vi "User Event Handle.vi"(8 "error in":errorcluster, 10 "Array 2":bool[](array[boolean])) -> (0 "error out":errorcluster)   [LabVIEW 2016]
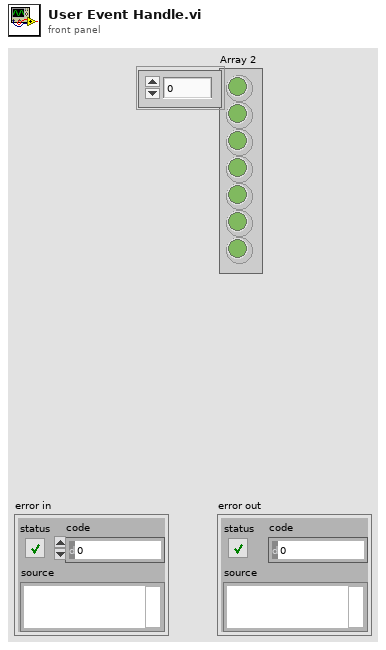
[diagram p1: front panel]
types:
  T1 = enum16{"Open", "Enqueue", "InsertQueue", "Release Queue", "Close"}
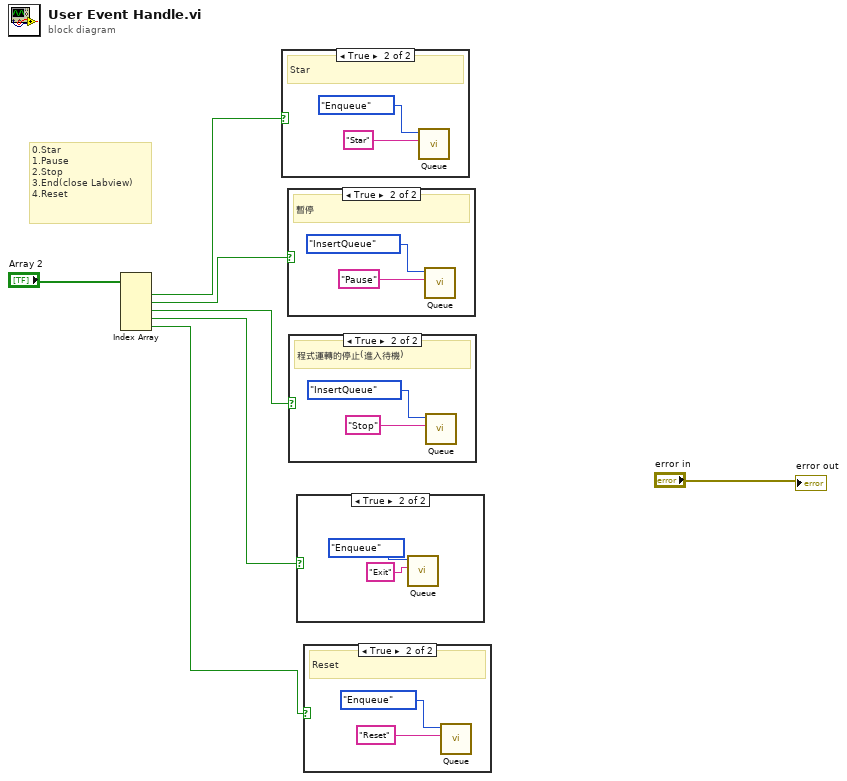
[diagram p0: block diagram]
diagram:
  # "0.Star\n1.Pause\n2.Stop\n3.End(close Labview)\n4.Reset"
  n1 = Index Array(array="Array 2") -> (element #1=w6:bool, element #2=w5:bool, element #3=w4:bool, element #4=w3:bool, element #5=w2:bool)  [unwired: 5 in]
  n2 = case shown="True" w6 {
    frame False {
    }
    frame True {
      # "Star"
      n3 = call "Queue.vi"("Message"="Star", "Function"=T1."Enqueue") -> ()  [unwired: 7 in, 3 out]
    }
  }
  n4 = case shown="True" w5 {
    frame False {
    }
    frame True {
      # "暫停"
      n5 = call "Queue.vi"("Message"="Pause", "Function"=T1."InsertQueue") -> ()  [unwired: 7 in, 3 out]
    }
  }
  n6 = case shown="True" w4 {
    frame False {
    }
    frame True {
      # "程式運轉的停止(進入待機)"
      n7 = call "Queue.vi"("Message"="Stop", "Function"=T1."InsertQueue") -> ()  [unwired: 7 in, 3 out]
    }
  }
  n8 = case shown="True" w3 {
    frame False {
    }
    frame True {
      n9 = call "Queue.vi"("Message"="Exit", "Function"=T1."Enqueue") -> ()  [unwired: 7 in, 3 out]
    }
  }
  n10 = case shown="True" w2 {
    frame False {
    }
    frame True {
      # "Reset"
      n11 = call "Queue.vi"("Message"="Reset", "Function"=T1."Enqueue") -> ()  [unwired: 7 in, 3 out]
    }
  }
  "error out" <- "error in"
